vi "Header Exists.vi"(8 "error in (no error)":errorcluster, 10 "header":string(combo)="User-Agent", 11 "HTTP Client Base in":refnum<class "HTTP Client Base.lvclass">) -> (0 "error out":errorcluster, 1 "value":string, 2 "header exists?":bool, 3 "HTTP Client Base out":refnum<class "HTTP Client Base.lvclass">)   [LabVIEW 2021, in "HTTP Client Base.lvclass"]
uses:
  HTTP Client Base.lvclass
  HTTP Client Base.lvclass/HTTP Client Base.ctl
  <vilib>/httpClient/LabVIEWHTTPClient.lvlib
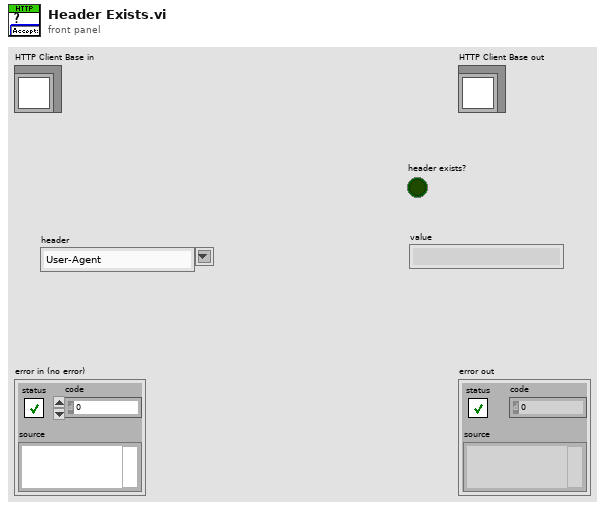
[diagram p1: front panel]
types:
  T1 = typedef "LabVIEWHTTPClient.lvlib/ClientHandle.ctl" = refnum<k1>
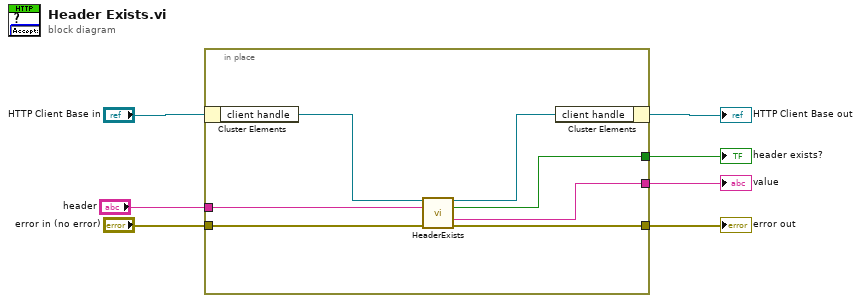
[diagram p0: block diagram]
diagram:
  n1 = in-place {
    in-place-border: "error in (no error)" -> [w14]
    in-place-border: [w13] -> w6
    in-place-border: "header" -> [w10]
    in-place-border: [w9] -> w3
    in-place-border: [w8] -> w1
    n2 = in-place-cluster #1("HTTP Client Base in") -> ("client handle"=w12:T1)
    n3 = call <vilib>:"HeaderExists.vi"("client handle"=w12, "header"=w10, "error in (no error)"=w14) -> ("client handle out"=w11:T1, "header exists?"=w8:bool, "value"=w9:string, "error out"=w13:errorcluster)  [unwired: 9 in]
    n4 = in-place-cluster #1("client handle"=w11) -> (→"HTTP Client Base out":refnum<class "HTTP Client Base.lvclass">)
  }
  "error out" <- w6
  "header exists?" <- w1
  "value" <- w3
